vi "HIOKI PW3390 Conf Sync source.vi"(0 "VISA Resource":refnum<visa-resource-name>, 1 "Set/Query (F: Set)":bool, 2 "CH (1)":i32=1 min=1 max=4, 5 "Sync Source (0: U1)":T2(ring), 11 "error in (no error)":errorcluster, 12 "OPC query (T: ON)":bool=TRUE, 13 "Error Out (F: Off)":bool) -> (4 "VISA Resource out":refnum<visa-resource-name>, 6 "Sync Source out":T1(ring), 15 "error out":errorcluster)   [LabVIEW 2009]
doc: "Set/Query\n Set: Send the setting commands for the device.\n Query: Query the setting of the device.\n\nSync Source\n Sets the Synchronized Source of the specified channel.\n\n<B>Note</B>\nThe settings for other channels in the measurement line combination will be changed.\nExt can be set only when the Motor Analysis Option is implemented and when CH B is set to Pulse."
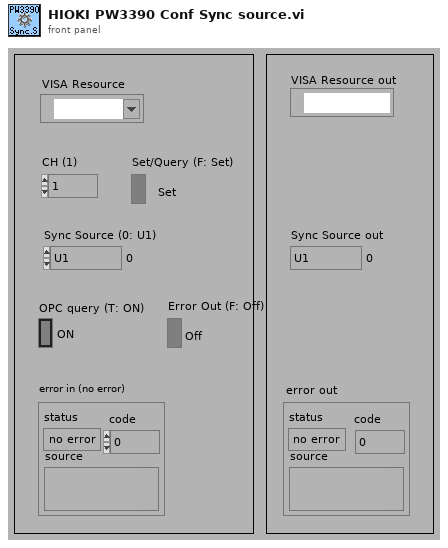
[diagram p1: front panel]
types:
  T1 = enum16{"U1", "U2", "U3", "U4", "I1", "I2", "I3", "I4", "Ext", "DC50ms", "DC100ms"}
  T2 = enum16{"U1", "U2", "U3", "U4", "I1", "I2", "I3", "I4", "EXT", "DC50ms", "DC100ms"}
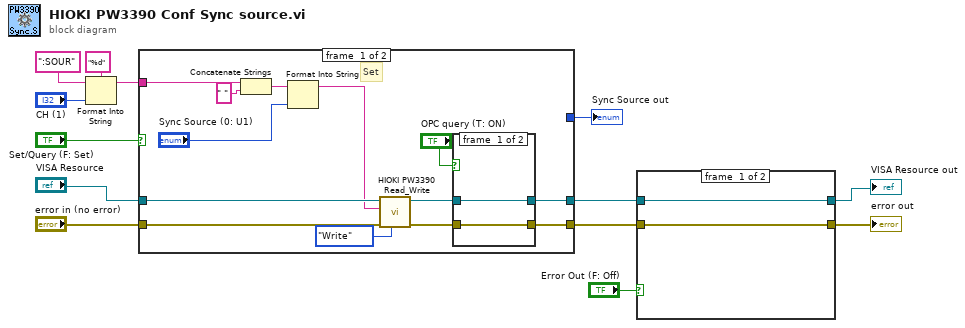
[diagram p0: block diagram]
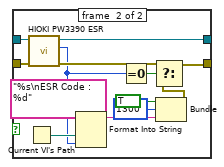
[diagram p2: hidden frame]
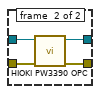
[diagram p3: hidden frame]
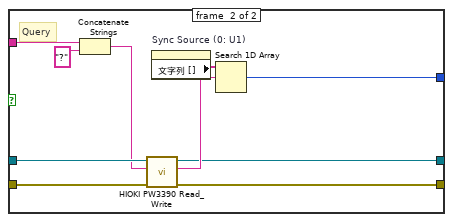
[diagram p4: hidden frame]
diagram:
  n1 = Format Into String(format string="%d", initial string=":SOUR", "CH (1)") -> (resulting string=w3:string)  [unwired: 1 in, 1 out]
  n2 = case shown="TRUE" "Set/Query (F: Set)" {
    tunnel: "error in (no error)" -> [w25 w41]
    tunnel: [w14 w36] -> w10
    tunnel: "VISA Resource" -> [w26 w42]
    tunnel: [w15 w37] -> w9
    tunnel: [_ w39] -> w7
    tunnel: w3 -> [w21 w35]
    frame #0 {
      # "Set"
      n3 = Concatenate Strings(w21, " " ("文字列")) -> (w20:string)
      n4 = Format Into String(initial string=w20, "Sync Source (0: U1)") -> (resulting string=w22:string)  [unwired: 2 in, 1 out]
      n5 = call <instrlib>:"HIOKI PW3390 Read_Write.vi"("Read/Write"=enum16{"Read", "Write"}."Write", "error in (no error)"=w25, "data in"=w22, "VISA Resource"=w26) -> ("error out"=w16:errorcluster, "VISA Resource out"=w17:refnum<visa-resource-name>)  [unwired: 5 in, 1 out]
      n6 = case shown="TRUE" "OPC query (T: ON)" {
        tunnel: [w28 w32] -> w15
        tunnel: [w27 w31] -> w14
        tunnel: w17 -> [w28 w30]
        tunnel: w16 -> [w27 w29]
        frame #0 {
        }
        frame #1 {
          n7 = call <instrlib>:"HIOKI PW3390 OPC.vi"("error in (no error)"=w29, "VISA Resource"=w30) -> ("error out"=w31:errorcluster, "VISA Resource out"=w32:refnum<visa-resource-name>)  [unwired: 7 in, 1 out]
        }
      }
    }
    frame #1 {
      # "Query"
      n8 = Concatenate Strings(w35, "?") -> (w33:string)
      n9 = call <instrlib>:"HIOKI PW3390 Read_Write.vi"("error in (no error)"=w41, "data in"=w33, "VISA Resource"=w42) -> ("error out"=w36:errorcluster, "data out"=w38:string, "VISA Resource out"=w37:refnum<visa-resource-name>)  [unwired: 6 in]
      n10 = property on="Sync Source (0: U1)" class="Enum （指定）"() -> ("文字列 []"=w40:string[])  [unwired: 2 in, 2 out]
      n11 = Search 1D Array(1D array=w40, element=w38) -> (index of element=w39:i32)  [unwired: 1 in]
    }
  }
  "Sync Source out" <- w7
  n12 = case shown="TRUE" "Error Out (F: Off)" {
    tunnel: w9 -> [w44 w57]
    tunnel: w10 -> [w43 w56]
    tunnel: [w43 w46] -> w8
    tunnel: [w44 w55] -> w1
    frame #0 {
    }
    frame #1 {
      n13 = Current VI's Path() -> (path=w53:path)
      n14 = call <instrlib>:"HIOKI PW3390 ESR.vi"("error in (no error)"=w56, "VISA Resource"=w57) -> ("error out"=w47:errorcluster, "Output Value"=w45:u8, "VISA Resource out"=w55:refnum<visa-resource-name>)  [unwired: 6 in, 1 out]
      n15 = Format Into String(format string="%s\nESR Code : %d", w53, w45) -> (resulting string=w49:string)  [unwired: 2 in, 1 out]
      n16 = Equal To 0?(x=w45) -> (x = 0?=w54:bool)
      n17 = Bundle("status"=TRUE, "code"=1300, w49) -> (w48:cluster{"status":bool, "code":i32, string})  [unwired: 1 in]
      n18 = Select(t=w47, s=w54, f=w48) -> (s? t:f=w46:errorcluster)
    }
  }
  "error out" <- w8
  "VISA Resource out" <- w1
